vi "Format TimeCol.vi"(10 "TimeFormat":u16(ring) caption="时间格式" items=["系统时间", "时间戳(s)"], 11 "Data":T1 {"Direction" items=["Tx", "Rx"]; "CANType" items=["CAN", "CANFD", "CANFD加速"]}) -> (3 "Time str":string)   [LabVIEW 2018, in "CAN FD.lvlib"]
uses:
  CAN FD.lvlib
  Typedef/CAN Data.ctl
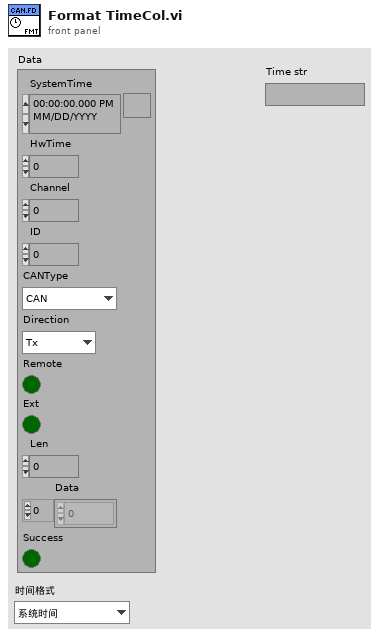
[diagram p1: front panel]
types:
  T1 = typedef "CAN FD.lvlib/CAN Data.ctl" = cluster{"SystemTime":timestamp, "HwTime":dbl, "Channel":u8, "ID":u32, "CANType":i16, "Direction":i16, "Remote":bool, "Ext":bool, "Len":u8, "Data":u8[], "Success":bool}
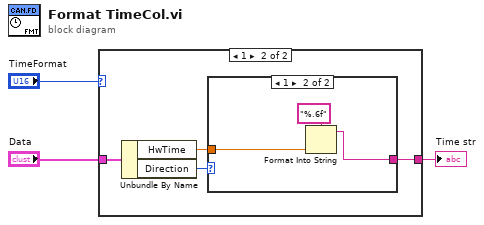
[diagram p0: block diagram]
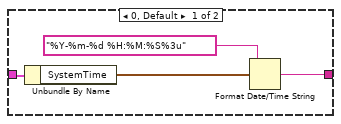
[diagram p2: hidden frame]
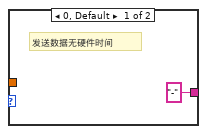
[diagram p3: hidden frame]
diagram:
  n1 = case shown="1" "TimeFormat" {
    tunnel: "Data" -> [w7 w11]
    tunnel: [w4 w8] -> w1
    frame 0, Default {
      n2 = Unbundle By Name(w7) -> ("SystemTime"=w6:timestamp)
      n3 = Format Date/Time String(time format string (%c)="%Y-%m-%d %H:%M:%S%3u" ("时间格式字符串(%c)"), seconds (now)=w6) -> (date/time string=w4:string)  [unwired: 1 in]
    }
    frame 1 {
      n4 = Unbundle By Name(w11) -> ("HwTime"=w9:dbl, "Direction"=w10:i16)
      n5 = case shown="1" w10 {
        tunnel: w9 -> [_ w15]
        tunnel: ["-" w13] -> w8
        frame 0, Default {
          # "发送数据无硬件时间"
        }
        frame 1 {
          n6 = Format Into String(format string="%.6f" ("格式字符串"), w15) -> (resulting string=w13:string)  [unwired: 2 in, 1 out]
        }
      }
    }
  }
  "Time str" <- w1
